vi "Generate_I2C.vi"(8 "Error_In":errorcluster, 10 "Mode":T1, 11 "I2C in":refnum<class "I2C.lvclass">) -> (0 "Error_Out":errorcluster, 3 "I2C out":refnum<class "I2C.lvclass">)   [LabVIEW 2021, in "I2C.lvclass"]
doc: "Parent class method for overriding"
uses:
  I2C.lvclass
  Controls/Mode.ctl
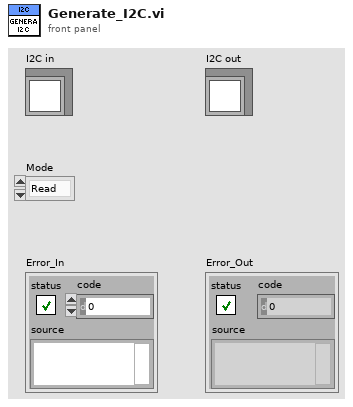
[diagram p1: front panel]
types:
  T1 = typedef "Mode.ctl" = enum16{"Read", "Write"}
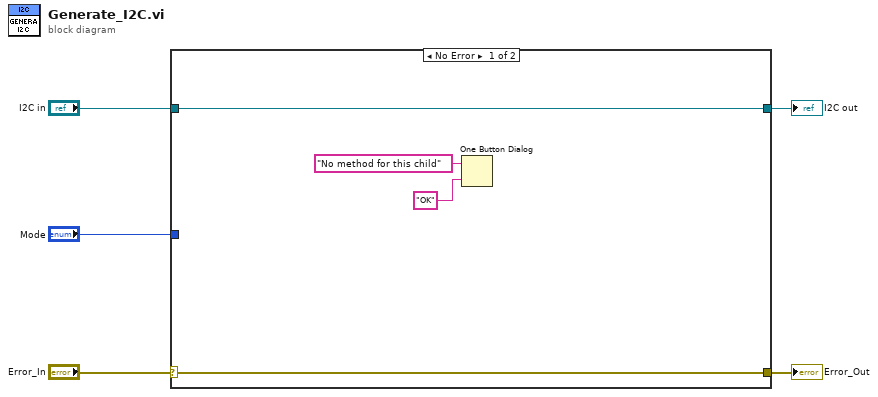
[diagram p0: block diagram]
diagram:
  n1 = case shown="No Error" "Error_In" {
    selector: "Error_In" -> [w8 w11]
    tunnel: [w8 w11] -> w4
    tunnel: [w9 w10] -> w2
    tunnel: "I2C in" -> [w9 w10]
    tunnel: "Mode" -> [_ _]
    frame No Error {
      n2 = One Button Dialog(message="No method for this child", button name ("OK")="OK") -> ()  [unwired: 1 out]
    }
    frame Error {
    }
  }
  "Error_Out" <- w4
  "I2C out" <- w2
